vi "key press sub.vi"(8 "Error In":errorcluster) -> (0 "Error Out":errorcluster, 1 "output cluster":T4, 2 "result":i32, 3 "keys pressed":T5(array[ring]))   [LabVIEW 2012]
uses:
  <vilib>/Utility/inputDevices.llb/keyboardAcquire.vi
  Downloads/Google Map - Multiple String Locations Example Folder/TypeDefs/Marker Labels.ctl
  Downloads/Google Map - Multiple String Locations Example Folder/TypeDefs/Marker Sizes.ctl
  Downloads/Google Map - Multiple String Locations Example Folder/TypeDefs/Map Types.ctl
panel:
  in  "System Stop Button":bool
  out "2D Picture":picture
  in  "Map Type":T1=enum."hybrid"
  in  "Refresh":bool
  in  "Marker Location Array":string[](array[string])=["11500 N Mo-Pac Expy Austin, TX 78759", "32 Watershaugh Rd, Warkworth, Northumberland, England", "38 Penny Green St Sugar Land TX", "Rannes St, Insch, Scotland"]
  in  "Color":u32(colorbox)=65793
  in  "Size":T2
  in  "Label":T3
  in  "Icon URL":string="http://lavag.org/public/style_extra/forum_imgs/LV.png"
  in  "Specify Icon?":bool=TRUE
  in  "Stop Button":bool
  out "Numeric Indicator 4":u8
  out "Numeric Indicator 3":u8
  out "Numeric Indicator 2":u8
  out "Numeric Indicator 1":u8
  # "Marker Customization"
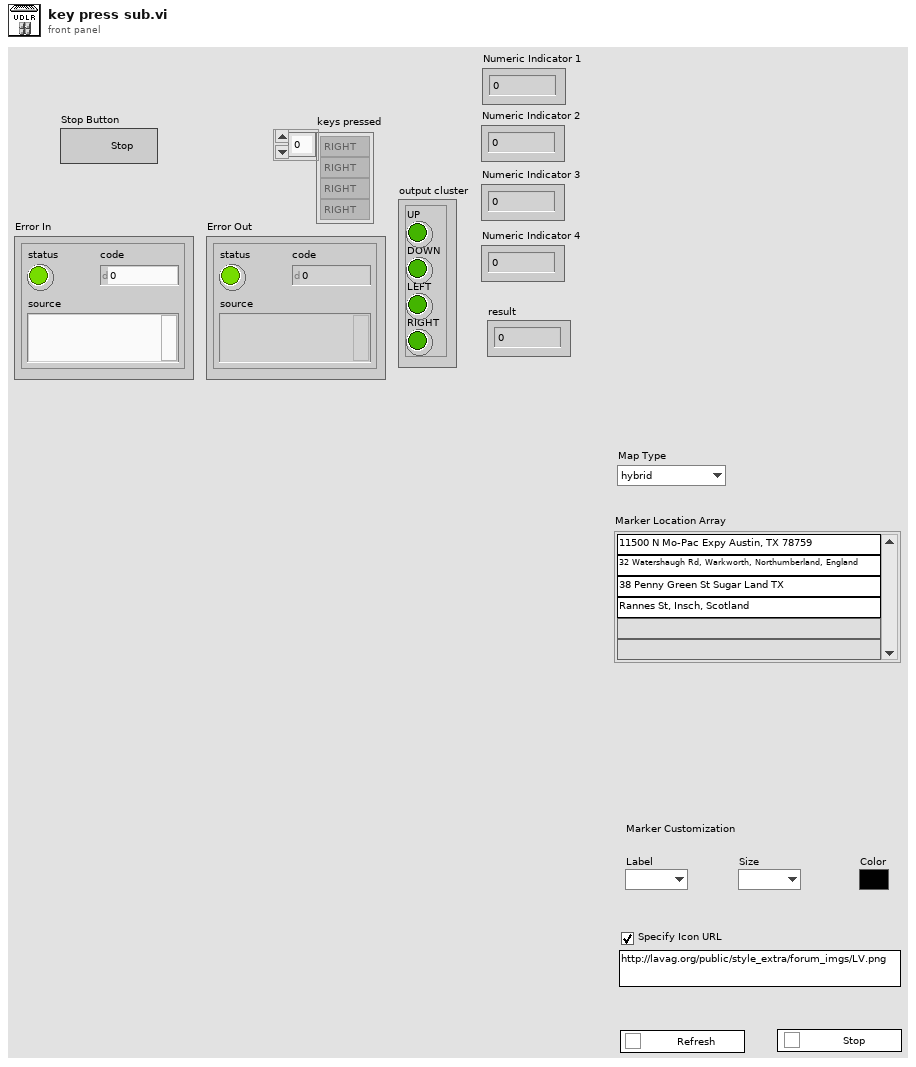
[diagram p1: front panel]
types:
  T1 = typedef "Map Types.ctl" = enum16{"roadmap", "satellite", "terrain", "hybrid"}
  T2 = typedef "Marker Sizes.ctl" = enum16{"", "small", "mid", "tiny"}
  T3 = typedef "Marker Labels.ctl" = enum16{"", "A", "B", "C", "D", "E", "F", "G", "H", "I", "J", "K", "M", "N", "O", "P", "Q", "R", "S", "T", "U", "V", "W", "X", "Y", "Z", "1", "2", "3", "4", "5", "6", "7", "8", "9", "0"}
  T4 = cluster{"UP":bool, "DOWN":bool, "LEFT":bool, "RIGHT":bool}
  T5 = enum16{"0", "1", "2", "3", "4", "5", "6", "7", "8", "9", "A", "B", "C", "D", "E", "F", "G", "H", "I", "J", "K", "L", "M", "N", "O", "P", "Q", "R", "S", "T", "U", "V", "W", "X", "Y", "Z", "F1", "F2", "F3", "F4", "F5", "F6", "F7", "F8", "F9", "F10", "F11", "F12", "F13", "F14", "F15", "ADD", "BACK", "BACKSLASH", "CAPITAL", "COMMA", "DECIMAL", "DELETE", "DIVIDE", "DOWN", "END", "EQUALS", "ESCAPE", "GRAVE (`)", "HOME", "INSERT", "LBRACKET", "LCONTROL", "LEFT", "L ALT", "LSHIFT", "LWIN", "MINUS", "MULTIPLY", "NEXT", "NUMLOCK", "NUMPAD_0", "NUMPAD_1", "NUMPAD_2", "NUMPAD_3", "NUMPAD_4", "NUMPAD_5", "NUMPAD_6", "NUMPAD_7", "NUMPAD_8", "NUMPAD_9", "PAUSE", "PERIOD", "PRIOR (PG UP)", "RBRACKET", "RCONTROL", "RETURN", "RIGHT", "R ALT", "RSHIFT", "RWIN", "SCROLL", "SEMICOLON", "SLASH", "SPACE", "SUBTRACT", "TAB", "UP", "ENTER (num pad)", "' (quote)"}[]
  T6 = enum16{"0", "1", "2", "3", "4", "5", "6", "7", "8", "9", "A", "B", "C", "D", "E", "F", "G", "H", "I", "J", "K", "L", "M", "N", "O", "P", "Q", "R", "S", "T", "U", "V", "W", "X", "Y", "Z", "F1", "F2", "F3", "F4", "F5", "F6", "F7", "F8", "F9", "F10", "F11", "F12", "F13", "F14", "F15", "ADD", "BACK", "BACKSLASH", "CAPITAL", "COMMA", "DECIMAL", "DELETE", "DIVIDE", "DOWN", "END", "EQUALS", "ESCAPE", "GRAVE (`)", "HOME", "INSERT", "LBRACKET", "LCONTROL", "LEFT", "L ALT", "LSHIFT", "LWIN", "MINUS", "MULTIPLY", "NEXT", "NUMLOCK", "NUMPAD_0", "NUMPAD_1", "NUMPAD_2", "NUMPAD_3", "NUMPAD_4", "NUMPAD_5", "NUMPAD_6", "NUMPAD_7", "NUMPAD_8", "NUMPAD_9", "PAUSE", "PERIOD", "PRIOR (PG UP)", "RBRACKET", "RCONTROL", "RETURN", "RIGHT", "R ALT", "RSHIFT", "RWIN", "SCROLL", "SEMICOLON", "SLASH", "SPACE", "SUBTRACT", "TAB", "UP", "ENTER (num pad)", "' (quote)"}
  T7 = typedef "LVBoundsTypeDef.ctl" = cluster{"Width":u32, "Height":u32}
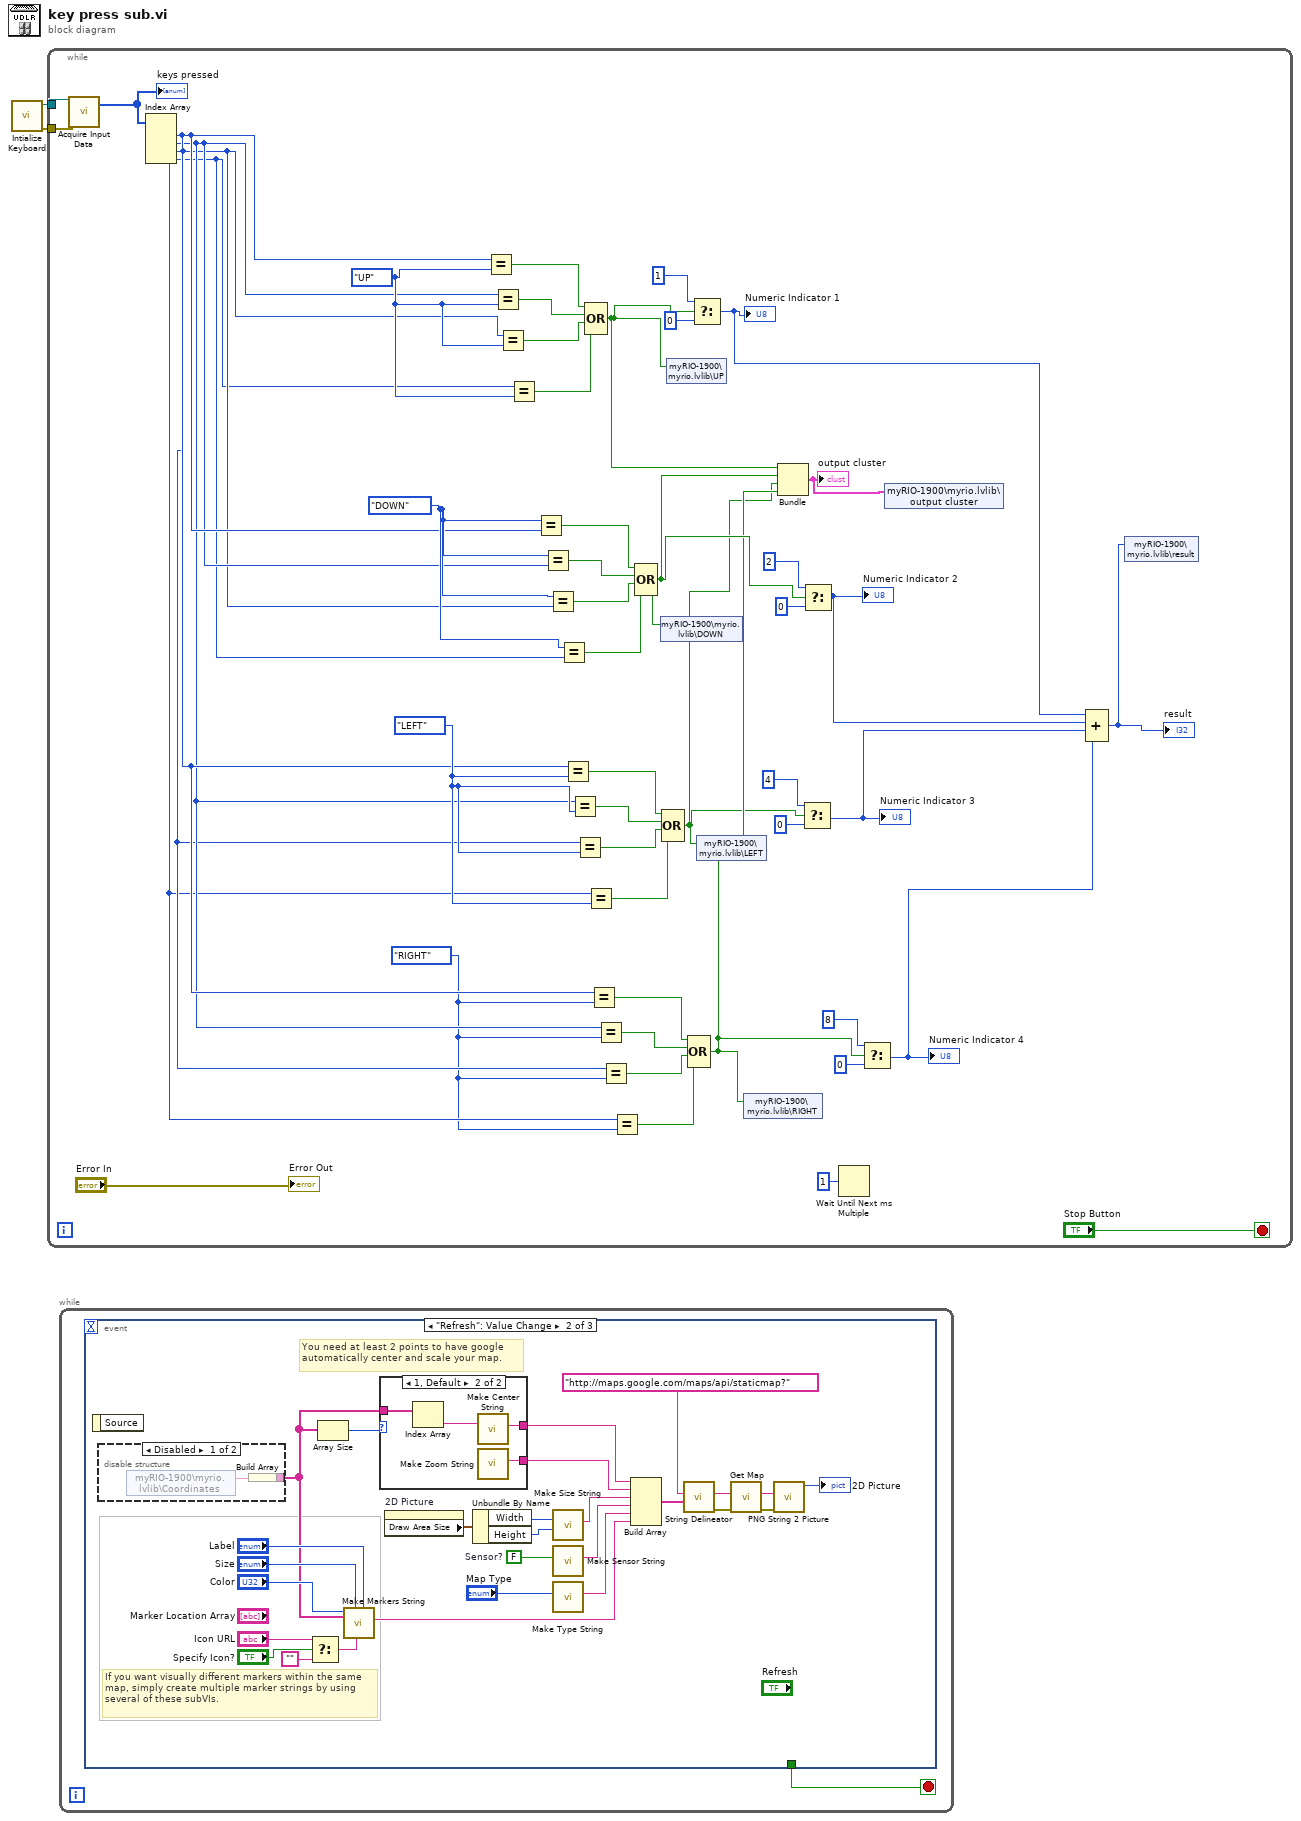
[diagram p0: block diagram]
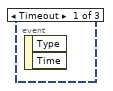
[diagram p2: hidden frame]
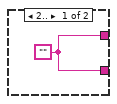
[diagram p4: hidden frame]
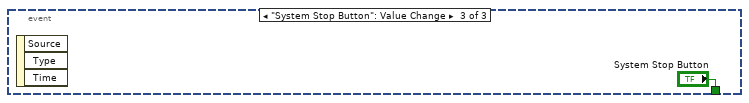
[diagram p5: hidden frame]
diagram:
  n1 = call <vilib>:"Intialize Keyboard.vi"() -> ("error out"=w2:errorcluster, "device ID"=w1:refnum<k1>)  [unwired: 10 in]
  n2 = while {
    tunnel: w2 -> [w13]
    tunnel: w1 -> [w12]
    stop <- "Stop Button" stop-if-true
    w27 = T6."RIGHT" ("element")
    w32 = T6."LEFT" ("element")
    w41 = T6."DOWN" ("element")
    w50 = T6."UP" ("element")
    n3 = call-poly <vilib>:"Acquire Input Data.vi"("device ID"=w12, "error in (no error)"=w13) -> ("keys pressed"=w14:T5)  [unwired: 15 in, 2 out]
    "keys pressed" <- w14
    n4 = Index Array(array=w14) -> (element #1=w31:T6, element #2=w30:T6, element #3=w29:T6, element #4=w28:T6)  [unwired: 4 in]
    n5 = Equal?(x=w31, y=w50) -> (x = y?=w49:bool)
    n6 = Equal?(x=w30, y=w50) -> (x = y?=w48:bool)
    n7 = Equal?(x=w29, y=w50) -> (x = y?=w47:bool)
    n8 = Equal?(x=w28, y=w50) -> (x = y?=w46:bool)
    n9 = Equal?(x=w41, y=w31) -> (x = y?=w42:bool)
    n10 = Equal?(x=w41, y=w30) -> (x = y?=w43:bool)
    n11 = Equal?(x=w41, y=w29) -> (x = y?=w44:bool)
    n12 = Equal?(x=w41, y=w28) -> (x = y?=w45:bool)
    n13 = Equal?(x=w31, y=w32) -> (x = y?=w40:bool)
    n14 = Equal?(x=w30, y=w32) -> (x = y?=w39:bool)
    n15 = Equal?(x=w29, y=w32) -> (x = y?=w38:bool)
    n16 = Compound Arithmetic op=OR(w49, w48, w47, w46) -> (w6:bool)
    n17 = Equal?(x=w28, y=w32) -> (x = y?=w37:bool)
    n18 = Equal?(x=w31, y=w27) -> (x = y?=w33:bool)
    n19 = Equal?(x=w30, y=w27) -> (x = y?=w34:bool)
    n20 = Equal?(x=w29, y=w27) -> (x = y?=w35:bool)
    n21 = Equal?(x=w28, y=w27) -> (x = y?=w36:bool)
    n22 = Compound Arithmetic op=OR(w42, w43, w44, w45) -> (w5:bool)
    n23 = shared-variable "myRIO-1900\\myrio.lvlib\\DOWN"(w5) -> ()  [unwired: 1 in, 1 out]
    n24 = Compound Arithmetic op=OR(w40, w39, w38, w37) -> (w3:bool)
    n25 = shared-variable "myRIO-1900\\myrio.lvlib\\UP"(w6) -> ()  [unwired: 1 in, 1 out]
    n26 = Compound Arithmetic op=OR(w33, w34, w35, w36) -> (w4:bool)
    n27 = Select(t=1, s=w6, f=0) -> (s? t:f=w18:i32)
    "Numeric Indicator 1" <- w18
    n28 = shared-variable "myRIO-1900\\myrio.lvlib\\LEFT"(w3) -> ()  [unwired: 1 in, 1 out]
    n29 = shared-variable "myRIO-1900\\myrio.lvlib\\RIGHT"(w4) -> ()  [unwired: 1 in, 1 out]
    n30 = Bundle(w6, w5, w3, w4) -> (w8:cluster{bool, bool, bool, bool})  [unwired: 1 in]
    "output cluster" <- w8
    n31 = Select(t=4, s=w3, f=0) -> (s? t:f=w16:i32)
    "Numeric Indicator 3" <- w16
    n32 = Select(t=2, s=w5, f=0) -> (s? t:f=w17:i32)
    "Numeric Indicator 2" <- w17
    n33 = Wait Until Next ms Multiple(millisecond multiple=u32 1) -> ()  [unwired: 1 out]
    n34 = Select(t=8, s=w4, f=0) -> (s? t:f=w15:i32)
    "Numeric Indicator 4" <- w15
    n35 = shared-variable "myRIO-1900\\myrio.lvlib\\output cluster"(w8) -> ()  [unwired: 1 in, 1 out]
    n36 = Compound Arithmetic op=ADD(w18, w17, w16, w15) -> (w7:i32)
    "result" <- w7
    n37 = shared-variable "myRIO-1900\\myrio.lvlib\\result"(w7) -> ()  [unwired: 1 in, 1 out]
    "Error Out" <- "Error In"
  }
  n38 = while {
    stop <- w51 stop-if-true
    n39 = event shown="[1] \"Refresh\": Value Change" {
      selector: _ -> [_ _ _]
      dyn-events: _ -> [_ _ _]
      timeout: _ -> [_ _ _]
      tunnel: [_ _ "System Stop Button"] -> w51
      event Timeout {
        n40 = event-data() -> ()  [unwired: 1 in, 2 out]
      }
      event "Refresh": Value Change {
        w65 = FALSE  # Sensor?
        # "You need at least 2 points to have google automatically center and scale your map."
        # "If you want visually different markers within the same map, simply create multiple marker strings by using several of these subVIs."
        n41 = event-data() -> ()  [unwired: 1 in, 1 out]
        n42 = disable-structure shown="Disabled" {
          disable-tunnel: [w79 _] -> w52
          frame Disabled {
            n43 = shared-variable "myRIO-1900\\myrio.lvlib\\Coordinates"() -> (w80:string)  [unwired: 1 in, 1 out]
            n44 = Build Array(w80) -> (w79:string[])
          }
          frame Enabled {
          }
        }
        n45 = Select(t="Icon URL", s="Specify Icon?", f="") -> (s? t:f=w54:string)
        n46 = Array Size(array=w52) -> (size(s)=w53:i32)
        n47 = call "Make Markers String.vi"("Label (optional)"="Label", "Icon URL (optional)"=w54, "Size (optional)"="Size", "Array of Locations"=w52, "Color (optional)"="Color") -> ("Markers string"=w76:string)  [unwired: 5 in, 1 out]
        n48 = case shown="1, Default" w53 {
          tunnel: [w81 w85] -> w77
          tunnel: [w81 w84] -> w78
          tunnel: w52 -> [_ w83]
          frame 2.. {
            w81 = ""
          }
          frame 1, Default {
            n49 = Index Array(array=w83) -> (element=w82:string)  [unwired: 1 in]
            n50 = call "Make Center String.vi"("Location string"=w82) -> ("Center string"=w85:string)  [unwired: 9 in, 1 out]
            n51 = call "Make Zoom String.vi"() -> ("Zoom string"=w84:string)  [unwired: 10 in, 1 out]
          }
        }
        n52 = property on="2D Picture" class="Pict"() -> ("Draw Area Size"=w71:T7)  [unwired: 2 in, 2 out]
        n53 = Unbundle By Name(w71) -> ("Width"=w72:u32, "Height"=w73:u32)
        n54 = call "Make Size String.vi"("Height (480)"=w73, "Width (480)"=w72) -> ("Size string"=w66:string)  [unwired: 8 in, 1 out]
        n55 = call "Make Sensor String.vi"("Sensor?"=w65) -> ("Sensor string"=w67:string)  [unwired: 9 in, 1 out]
        n56 = call "Make Type String.vi"("Map Type"="Map Type") -> ("maptype string"=w69:string)  [unwired: 9 in, 1 out]
        n57 = Build Array(w77, w78, w66, w67, w69, w76) -> (w68:string[])
        n58 = call "String Delineator.vi"("Array of Strings"=w68, "Base String"="http://maps.google.com/maps/api/staticmap?" ("URL")) -> ("error in (no error)"=w74:errorcluster, "New String"=w75:string)  [unwired: 8 in]
        n59 = call "Get Map.vi"("error in (no error)"=w74, "URL"=w75) -> ("error out"=w63:errorcluster, "Body"=w62:string)  [unwired: 8 in]
        n60 = call "PNG String 2 Picture.vi"("error in (no error)"=w63, "PNG Data as String"=w62) -> ("Picture Out"=→"2D Picture":picture)  [unwired: 8 in, 1 out]
      }
      event "System Stop Button": Value Change {
        n61 = event-data() -> ()  [unwired: 1 in, 3 out]
      }
    }
  }
